vi "Get NHMFL Synth Object.vi"() -> (3 "Module":refnum<class "Template Module.lvclass">)   [LabVIEW 2016]
uses:
  Measure_core/Template Module/Template Module.lvclass
  NHMFL Synthesizer.lvclass
  C:/github/Measure_core/Template Module/Template Module.lvclass
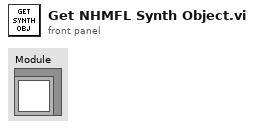
[diagram p1: front panel]
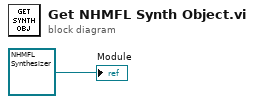
[diagram p0: block diagram]
diagram:
  "Module" <- refnum<class "NHMFL Synthesizer.lvclass"> refnum ("NHMFL Synthesizer.lvclass")
